vi "Mask Write Holding Register.vi"(4 "OR mask":u16, 6 "AND mask":u16, 8 "error in (no error)":errorcluster, 10 "address":u16, 11 "device data model in":refnum<class "Standard Data Model.lvclass">) -> (0 "error out":errorcluster, 3 "device data model out":refnum<class "Standard Data Model.lvclass">)   [LabVIEW 2017, in "SubVIs.lvlib" / "Standard Data Model.lvclass"]
doc: "Writes the masked value of a single register using an <b>AND mask</b> and an <b>OR mask</b> using the equation below:\nResult=(Current Value AND AndMask) OR (OrMask AND !AndMask)"
uses:
  <vilib>/Modbus/subvis/Data and Functions/Standard Data Model/Standard Data Model.lvclass
  <vilib>/Modbus/subvis/Data and Functions/Standard Data Model/Standard Data Model.lvclass/Standard Data Model.ctl
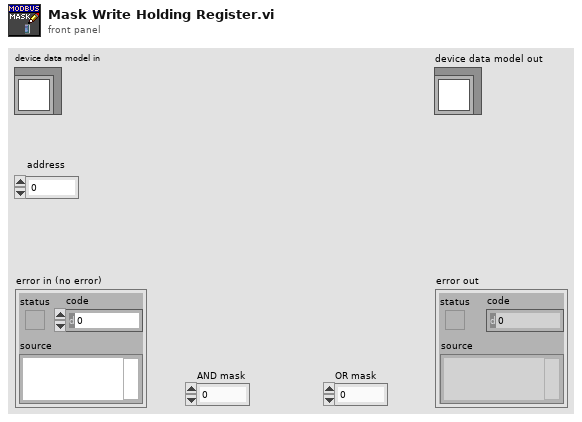
[diagram p1: front panel]
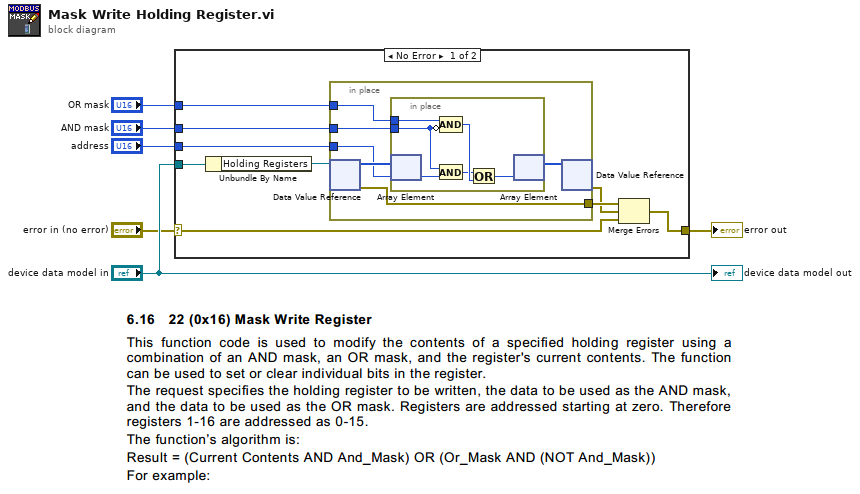
[diagram p0: block diagram]
diagram:
  n1 = case shown="No Error" "error in (no error)" {
    selector: "error in (no error)" -> [w7 w28]
    tunnel: "device data model in" -> [w15 _]
    tunnel: [w14 w28] -> w5
    tunnel: "address" -> [w12 _]
    tunnel: "AND mask" -> [w11 _]
    tunnel: "OR mask" -> [w10 _]
    frame No Error {
      n2 = Unbundle By Name(w15) -> ("Holding Registers"=w13:refnum<data-value>)
      n3 = in-place {
        in-place-border: w12 -> [w20]
        in-place-border: w11 -> [w18]
        in-place-border: w10 -> [w17]
        in-place-border: [w16] -> w9
        n4 = in-place-dvr #1(w13) -> (w21:u16[], w16:errorcluster)
        n5 = in-place {
          in-place-border: w18 -> [w22]
          in-place-border: w17 -> [w24]
          n6 = in-place-array #2(w21, w20) -> (w23:u16)
          n7 = And(x=w22, y=w23) -> (x .and. y?=w26:u16)
          n8 = Compound Arithmetic op=AND(w24, invert w22) -> (w27:u16)
          n9 = Or(x=w26, y=w27) -> (x .or. y?=w25:u16)
          n10 = in-place-array #2(w25) -> (w19:u16[])  [unwired: 1 out]
        }
        n11 = in-place-dvr #1(w19) -> (w8:errorcluster)  [unwired: 1 out]
      }
      n12 = Merge Errors(w9, w8, w7) -> (w14:errorcluster)
    }
    frame Error {
    }
  }
  "error out" <- w5
  "device data model out" <- "device data model in"
